vi "FIR_4Decimate_FilterBank.vi"(8 "data valid in":bool, 9 "Q in":fxp<+/-,16,14>[](array[numeric])=[0.0, 0.0, 0.0, 0.0], 10 "I in":fxp<+/-,16,14>[](array[numeric])=[0.0, 0.0, 0.0, 0.0]) -> (0 "data valid out":bool, 1 "Q out":fxp<+/-,16,14>, 2 "I out":fxp<+/-,16,14>)   [LabVIEW 2013]
uses:
  <vilib>/rvi/FXPMathLib/FxpConvert/subVIs/nifxpmath_Convert_SimConfig.ctl
  <vilib>/fxp/LVFixedPointQuantizationPolicyTypeDef.ctl
  <vilib>/fxp/LVFixedPointOverflowPolicyTypeDef.ctl
  <vilib>/rvi/FXPMathLib/FxpConvert/simVIs/DllFxpConvertTemp_sub.vi
  <vilib>/rvi/FXPMathLib/FxpInterpret/XNode/nifxpmath_Interpret.xnode
  <vilib>/rvi/FXPMathLib/FxpConvert/XNode/nifxpmath_Convert.xnode
  <vilib>/rvi/FXPMathLib/FxpAdd/XNode/nifxpmath_Add.xnode
  <vilib>/rvi/FXPMathLib/sim/FxpSim.dll
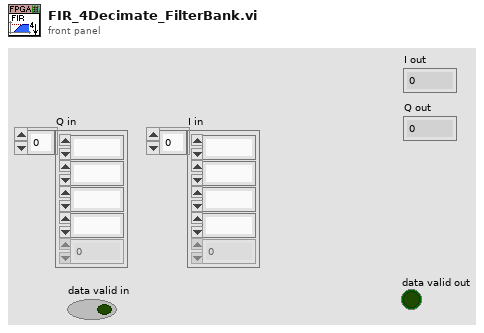
[diagram p1: front panel]
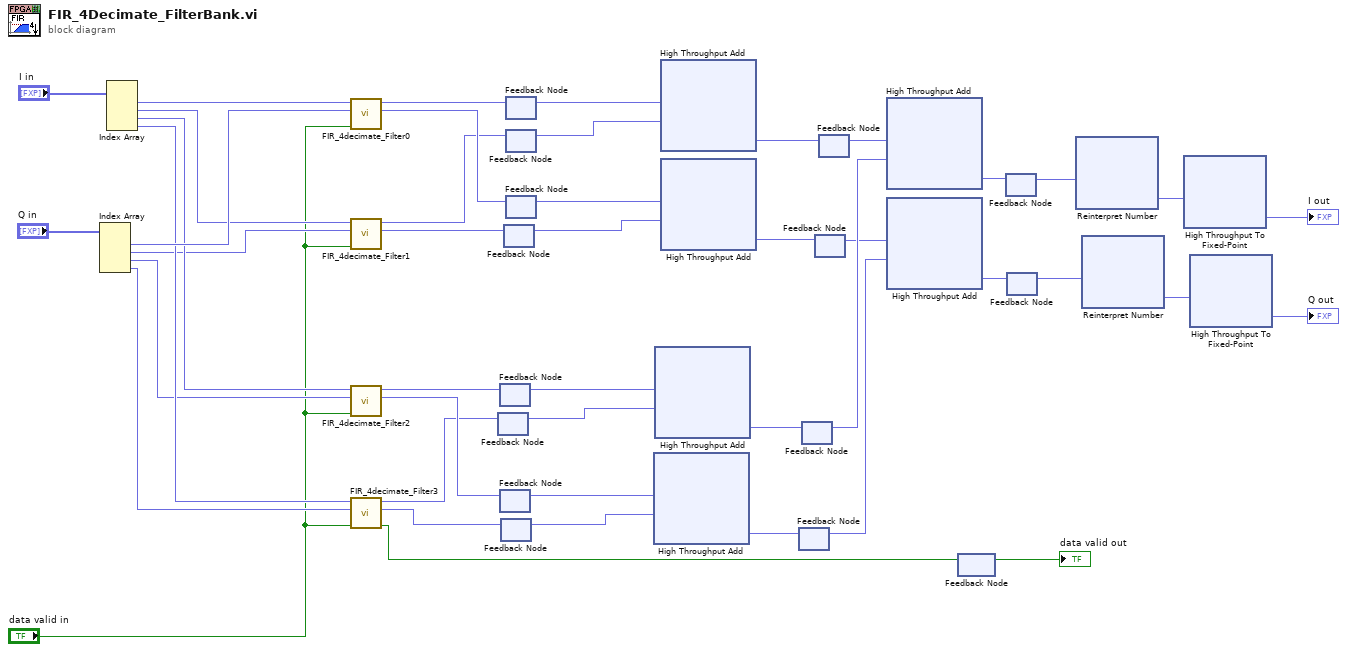
[diagram p0: block diagram]
diagram:
  n1 = Index Array(array="Q in") -> (element #1=w24:fxp<+/-,16,14>, element #2=w19:fxp<+/-,16,14>, element #3=w18:fxp<+/-,16,14>, element #4=w17:fxp<+/-,16,14>)  [unwired: 4 in]
  n2 = Index Array(array="I in") -> (element #1=w27:fxp<+/-,16,14>, element #2=w22:fxp<+/-,16,14>, element #3=w21:fxp<+/-,16,14>, element #4=w20:fxp<+/-,16,14>)  [unwired: 4 in]
  n3 = call "FIR_4decimate_Filter0.vi"("valid in"="data valid in", "Q in"=w24, "I in"=w27) -> ("Q out"=w15:fxp<+/-,16,14>, "I out"=w23:fxp<+/-,16,14>)  [unwired: 6 in, 1 out]
  n4 = call "FIR_4decimate_Filter1.vi"("valid in"="data valid in", "Q in"=w19, "I in"=w22) -> ("Q out"=w13:fxp<+/-,16,14>, "I out"=w14:fxp<+/-,16,14>)  [unwired: 6 in, 1 out]
  n5 = call "FIR_4decimate_Filter2.vi"("valid in"="data valid in", "Q in"=w18, "I in"=w21) -> ("Q out"=w11:fxp<+/-,16,14>, "I out"=w12:fxp<+/-,16,14>)  [unwired: 6 in, 1 out]
  n6 = call "FIR_4decimate_Filter3.vi"("valid in"="data valid in", "Q in"=w17, "I in"=w20) -> ("valid out"=w8:bool, "Q out"=w9:fxp<+/-,16,14>, "I out"=w10:fxp<+/-,16,14>)  [unwired: 6 in]
  n7 = feedback #1() -> (w42:fxp<+/-,16,14>)  [unwired: 1 in]
  n8 = feedback-in #1(w10) -> ()
  n9 = feedback #2() -> (w43:fxp<+/-,16,14>)  [unwired: 1 in]
  n10 = feedback-in #2(w12) -> ()
  n11 = feedback #3() -> (w40:fxp<+/-,16,14>)  [unwired: 1 in]
  n12 = feedback-in #3(w11) -> ()
  n13 = feedback #4() -> (w41:fxp<+/-,16,14>)  [unwired: 1 in]
  n14 = feedback-in #4(w9) -> ()
  n15 = feedback #5() -> (w38:fxp<+/-,16,14>)  [unwired: 1 in]
  n16 = feedback-in #5(w13) -> ()
  n17 = feedback #6() -> (w45:fxp<+/-,16,14>)  [unwired: 1 in]
  n18 = feedback-in #6(w23) -> ()
  n19 = feedback #7() -> (w44:fxp<+/-,16,14>)  [unwired: 1 in]
  n20 = feedback-in #7(w14) -> ()
  n21 = feedback #8() -> (w39:fxp<+/-,16,14>)  [unwired: 1 in]
  n22 = feedback-in #8(w15) -> ()
  n23 = xnode ("High Throughput Add")("x"=w40, "y"=w41) -> ("x+y"=w28:fxp<+/-,19,15>)
  n24 = xnode ("High Throughput Add")("x"=w43, "y"=w42) -> ("x+y"=w33:fxp<+/-,19,15>)
  n25 = xnode ("High Throughput Add")("x"=w45, "y"=w44) -> ("x+y"=w34:fxp<+/-,19,15>)
  n26 = xnode ("High Throughput Add")("x"=w39, "y"=w38) -> ("x+y"=w29:fxp<+/-,19,15>)
  n27 = feedback #9() -> (w30:fxp<+/-,19,15>)  [unwired: 1 in]
  n28 = feedback-in #9(w28) -> ()
  n29 = feedback #10() -> (w37:fxp<+/-,19,15>)  [unwired: 1 in]
  n30 = feedback-in #10(w33) -> ()
  n31 = feedback #11() -> (w31:fxp<+/-,19,15>)  [unwired: 1 in]
  n32 = feedback-in #11(w29) -> ()
  n33 = feedback #12() -> (w36:fxp<+/-,19,15>)  [unwired: 1 in]
  n34 = feedback-in #12(w34) -> ()
  n35 = xnode ("High Throughput Add")("x"=w36, "y"=w37) -> ("x+y"=w35:fxp<+/-,20,16>)
  n36 = xnode ("High Throughput Add")("x"=w31, "y"=w30) -> ("x+y"=w32:fxp<+/-,20,16>)
  n37 = feedback #13() -> (→"data valid out":bool)  [unwired: 1 in]
  n38 = feedback-in #13(w8) -> ()
  n39 = feedback #14() -> (w5:fxp<+/-,20,16>)  [unwired: 1 in]
  n40 = feedback-in #14(w35) -> ()
  n41 = feedback #15() -> (w2:fxp<+/-,20,16>)  [unwired: 1 in]
  n42 = feedback-in #15(w32) -> ()
  n43 = xnode "Reinterpret Number"("x"=w5) -> ("y"=w6:fxp<+/-,20,14>)
  n44 = xnode "Reinterpret Number"("x"=w2) -> ("y"=w3:fxp<+/-,20,14>)
  n45 = xnode ("High Throughput To Fixed-Point")("x"=w6) -> ("y"=→"I out":fxp<+/-,16,14>)
  n46 = xnode ("High Throughput To Fixed-Point")("x"=w3) -> ("y"=→"Q out":fxp<+/-,16,14>)
